vi "View Artist Library Request.vi"(8 "error in (no error)":errorcluster, 11 "MusicManagerActor in":refnum<class "MusicManagerActor.lvclass">) -> (0 "error out":errorcluster, 3 "MusicManagerActor out":refnum<class "MusicManagerActor.lvclass">)   [LabVIEW 2015, in "MusicManagerActor.lvlib" / "MusicManagerActor.lvclass"]
uses:
  MusicManagerActor.lvclass
  MusicManagerActor.lvclass/MusicManagerActor.ctl
  SongBrowserActor/SongBrowserActor Messages/Display Artist Library Msg/Display Artist Library Msg.lvclass
  SongQueueActor/SongQueueActor Messages/Set Visibility Of Queue List Msg/Set Visibility Of Queue List Msg.lvclass
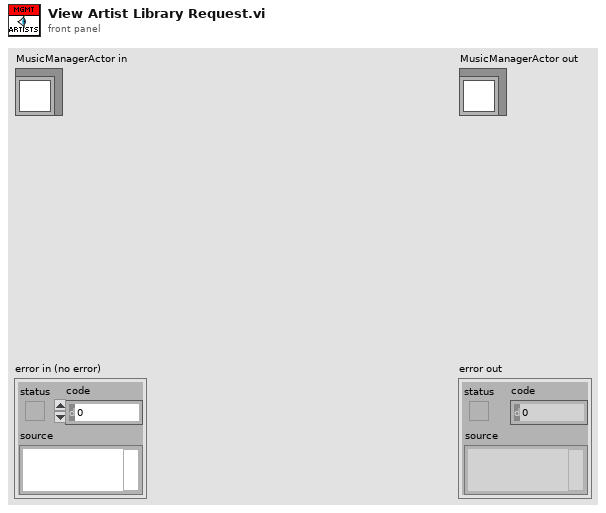
[diagram p1: front panel]
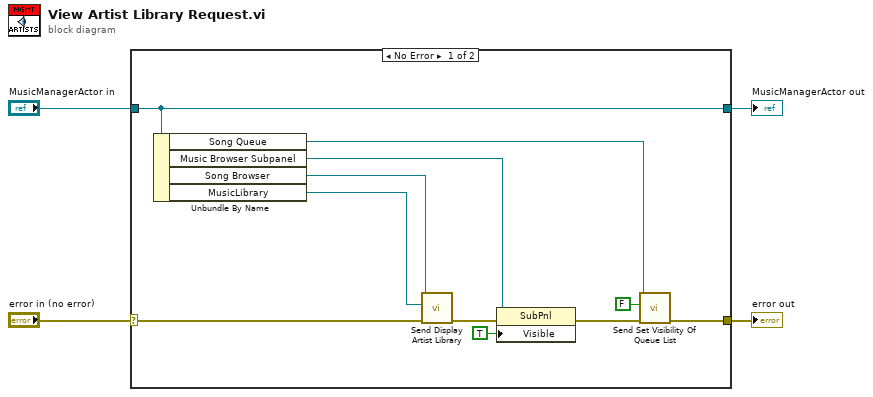
[diagram p0: block diagram]
diagram:
  n1 = case shown="No Error" "error in (no error)" {
    selector: "error in (no error)" -> [w13 w17]
    tunnel: [w5 w17] -> w3
    tunnel: [w15 w16] -> w1
    tunnel: "MusicManagerActor in" -> [w15 w16]
    frame No Error {
      n2 = Unbundle By Name(w15) -> ("Song Queue"=w7:refnum<class "Message Enqueuer.lvclass">, "Music Browser Subpanel"=w9:refnum<vi>, "Song Browser"=w12:refnum<class "Message Enqueuer.lvclass">, "MusicLibrary"=w14:refnum<class "MusicLibrary.lvclass">)
      n3 = call "Send Display Artist Library.vi"("error in (no error)"=w13, "MusicLibrary"=w14, "Message Enqueuer in"=w12) -> ("error out"=w10:errorcluster)  [unwired: 7 in, 1 out]
      n4 = property class="SubPnl"(reference=w9, error in=w10, "Visible"=TRUE) -> (error out=w6:errorcluster)  [unwired: 1 out]
      n5 = call "Send Set Visibility Of Queue List.vi"("error in (no error)"=w6, "Visible"=FALSE, "Message Enqueuer in"=w7) -> ("error out"=w5:errorcluster)  [unwired: 7 in, 1 out]
    }
    frame Error {
    }
  }
  "error out" <- w3
  "MusicManagerActor out" <- w1
